vi "Read Value (SubVI).vi"(0 "ILabVIEW In":refnum<k24>, 1 "DeviceType":i32(ring) items=["Controller", "RUI", "PC", "CommsCard"], 2 "Zone":i32, 3 "ParameterID":dbl, 4 "InstanceId":i32, 5 "error in (no error)":errorcluster, 6 "TemperatureUnits":u8(ring) items=["Degrees F", "Degrees C"]) -> (14 "ILabVIEW Out":refnum<k24>, 17 "Value Out":string, 19 "error out":errorcluster)   [LabVIEW 2017]
doc: "by Tanguy BOULARD"
uses:
  dll/Watbus.dll
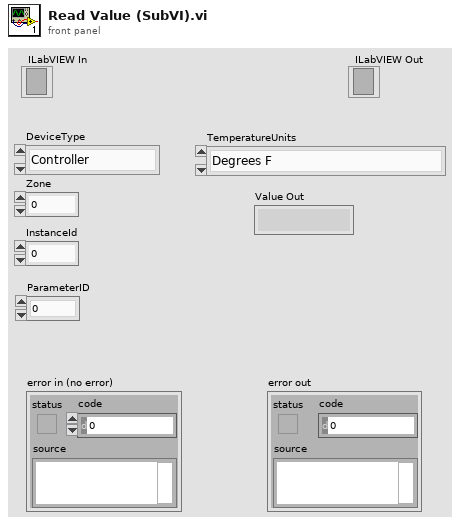
[diagram p1: front panel]
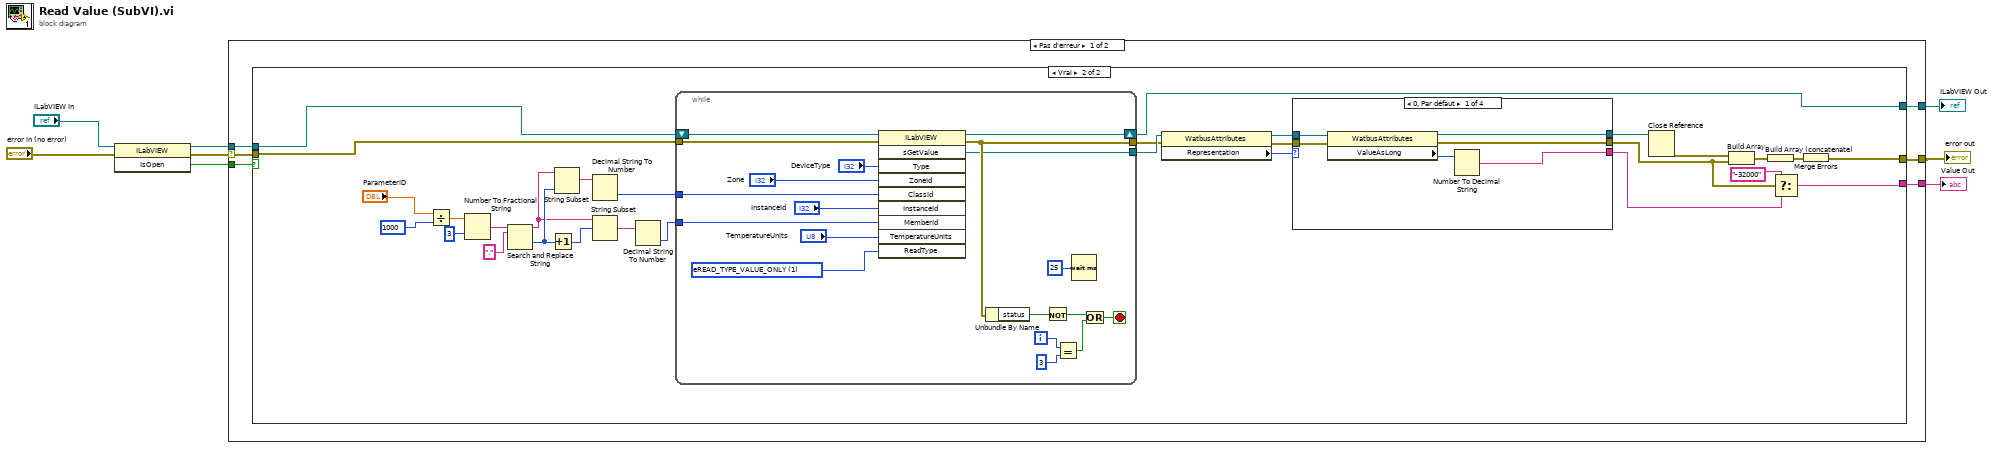
[diagram p0: block diagram]
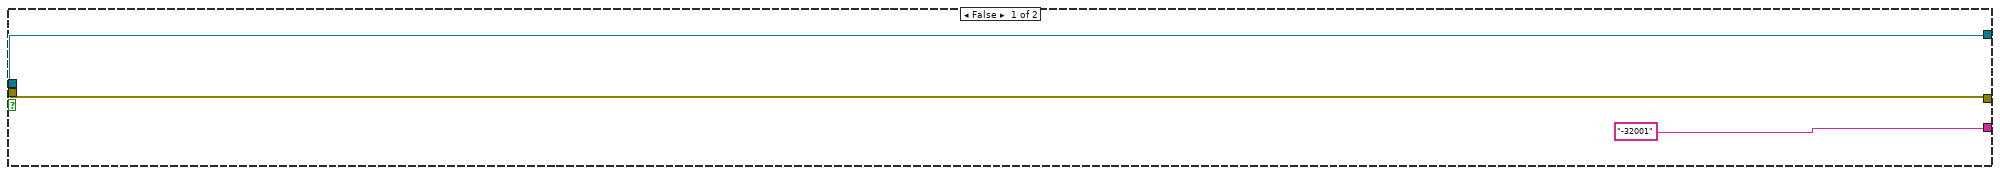
[diagram p2: hidden frame]
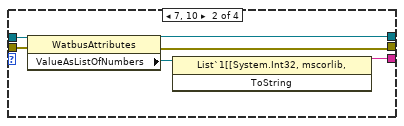
[diagram p3: hidden frame]
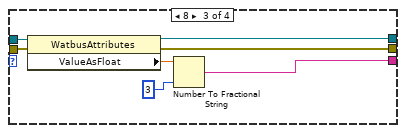
[diagram p4: hidden frame]
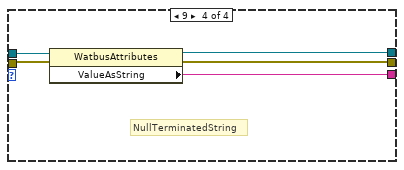
[diagram p5: hidden frame]
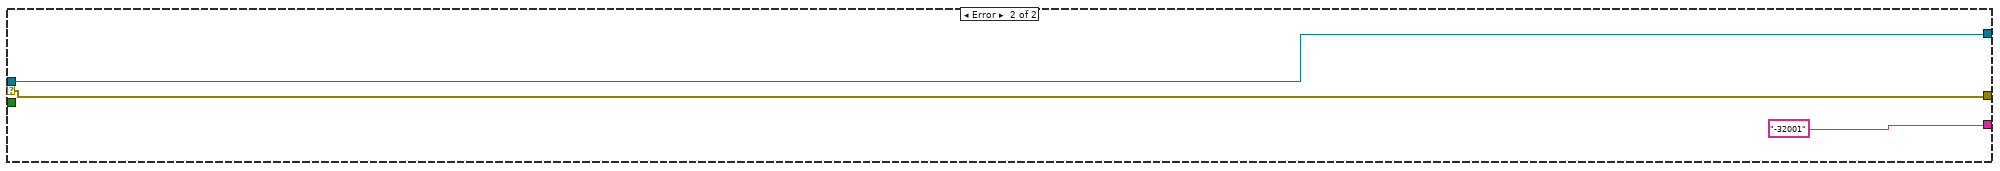
[diagram p6: hidden frame]
diagram:
  n1 = invoke class="ILabVIEW" method="IsOpen"(reference="ILabVIEW In", error in="error in (no error)") -> (reference out=w2:refnum<k24>, error out=w7:errorcluster, "IsOpen"=w5:bool)  [unwired: 1 in]
  n2 = case shown="Pas d'erreur" w7 {
    selector: w7 -> [w10 w93]
    tunnel: [w14 "-32001" ("ValueAsString")] -> w8
    tunnel: [w13 w91] -> w3
    tunnel: w2 -> [w12 w91]
    tunnel: [w11 w93] -> w1
    tunnel: w5 -> [w9 _]
    frame No Error {
      n3 = case shown="Vrai" w9 {
        tunnel: ["-32001" ("ValueAsString") w42] -> w14
        tunnel: w12 -> [w16 w47]
        tunnel: w10 -> [w15 w46]
        tunnel: [w15 w45] -> w11
        tunnel: [w16 w43] -> w13
        frame False {
        }
        frame True {
          n4 = Divide(x="ParameterID", y=1000) -> (x/y=w31:dbl)
          n5 = Number To Fractional String(number=w31, precision (6)=i16 3) -> (F-format string=w19:string)  [unwired: 2 out]
          n6 = Search and Replace String(input string=w19, search string=".") -> (result string=w18:string, offset past replacement=w36:i32)  [unwired: 1 in, 7 out]
          n7 = Increment(x=w36) -> (x+1=w34:i32)
          n8 = String Subset(string=w18, length (rest)=w36) -> (substring=w37:string)  [unwired: 1 out]
          n9 = Decimal String To Number(string=w37) -> (number=w29:i32)  [unwired: 3 out]
          n10 = String Subset(string=w18, offset (0)=w34) -> (substring=w35:string)  [unwired: 1 out]
          n11 = Decimal String To Number(string=w35) -> (number=w28:i32)  [unwired: 3 out]
          n12 = while {
            tunnel: [w48] -> w41
            tunnel: w29 -> [w66]
            tunnel: w28 -> [w65]
            shift-right: [w62] -> w43
            shift-left: w47 -> [w64]
            tunnel: w46 -> [w63]
            tunnel: [w58] -> w20
            i -> [w54]
            stop <- w55 stop-if-true
            w49 = u8 1 items=["eREAD_TYPE_VALUE_ONLY"=1, "eREAD_TYPE_VALUE_AND_ATTRIBUTES"=2] ("ReadType")
            n13 = invoke class="ILabVIEW" method="sGetValue"(reference=w64, error in=w63, "Type"="DeviceType", "ZoneId"="Zone", "ClassId"=w66, "InstanceId"="InstanceId", "MemberId"=w65, "TemperatureUnits"="TemperatureUnits", "ReadType"=w49) -> (reference out=w62:refnum<k24>, error out=w58:errorcluster, "sGetValue"=w48:refnum<k24>)  [unwired: 1 in, 7 out]
            n14 = Unbundle By Name(w58) -> ("status"=w57:bool)
            n15 = Not(x=w57) -> (.not. x?=w56:bool)
            n16 = Equal?(x=w54, y=3) -> (x = y?=w53:bool)
            n17 = Wait (ms)(milliseconds to wait=u32 25) -> ()  [unwired: 1 out]
            n18 = Or(x=w56, y=w53) -> (x .or. y?=w55:bool)
          }
          n19 = property class="WatbusAttributes"(reference=w41, error in=w20) -> (reference out=w40:refnum<k24>, error out=w38:errorcluster, "Representation"=w39:i32)
          n20 = case shown="0, Par défaut" w39 {
            tunnel: w40 -> [w72 w78 w85 w90]
            tunnel: [w70 w76 w83 w87] -> w26
            tunnel: w38 -> [w69 w75 w81 w89]
            tunnel: [w68 w74 w80 w88] -> w23
            tunnel: [w67 w73 w79 w86] -> w25
            frame 0, Default {
              n21 = property class="WatbusAttributes"(reference=w72, error in=w69) -> (reference out=w67:refnum<k24>, error out=w68:errorcluster, "ValueAsLong"=w71:i64)
              n22 = Number To Decimal String(number=w71) -> (decimal integer string=w70:string)  [unwired: 1 out]
            }
            frame 7, 10 {
              n23 = property class="WatbusAttributes"(reference=w78, error in=w75) -> (reference out=w73:refnum<k24>, error out=w74:errorcluster, "ValueAsListOfNumbers"=w77:refnum<k24>)
              n24 = invoke class="List`1[[System.Int32, mscorlib," method="ToString"(reference=w77) -> ("ToString"=w76:string)  [unwired: 2 in, 2 out]
            }
            frame 8 {
              n25 = property class="WatbusAttributes"(reference=w85, error in=w81) -> (reference out=w79:refnum<k24>, error out=w80:errorcluster, "ValueAsFloat"=w84:sgl)
              n26 = Number To Fractional String(number=w84, precision (6)=i16 3) -> (F-format string=w83:string)  [unwired: 2 out]
            }
            frame 9 {
              # "NullTerminatedString"
              n27 = property class="WatbusAttributes"(reference=w90, error in=w89) -> (reference out=w86:refnum<k24>, error out=w88:errorcluster, "ValueAsString"=w87:string)
            }
          }
          n28 = Close Reference(reference=w25) -> (error out=w24:errorcluster)  [unwired: 1 in]
          n29 = Build Array(w24, w23) -> (w22:errorcluster[])
          n30 = Build Array (concatenate)(w22) -> (w21:errorcluster[])
          n31 = Select(t="-32000" ("ValueAsString"), s=w23, f=w26) -> (s? t:f=w42:string)
          n32 = Merge Errors(w21) -> (w45:errorcluster)
        }
      }
    }
    frame Error {
    }
  }
  "error out" <- w1
  "Value Out" <- w8
  "ILabVIEW Out" <- w3
